vi "Agilent 34970 EZ Scan-AJ Version.vi"() -> ()   [LabVIEW 2018]
doc: "This Example VI shows how to set up the scan list and then take a measurement. This VI uses the EZ measurement VIs. These VIs offer the quickest and easiest use. However, they do not let you have different types of measurements in the same scan list. For a full description of the three ways to setup and scan using the HP34970A, read the text below.\n\nAlthough this driver only shows Current and Frequency (for simplicity), there are EZ Measurement VIs for all six measurement types.\n\n====================\nSetting up and performing a scan\n====================\nThe HP34970A provides commands for setting up a scan in three ways that differ in their complexity and the amount of control offered:\n\n1. Advanced:\nEvery aspect of the measurement, scan, scan list, and read is put in a different command to allow the greatest flexibility. For example, using the advanced configure VIs, you can set up a scan list consisting of different measurement types on different channels. The \"HP34970A Advanced Scan Example.vi\" demonstrates usage of these VIs.\n\n2. Medium:\nThe instrument also offers a command that wraps up configuring individual channels and the scan list. This is represented in the driver by \"HP34970A Conf EZ.vi\". This driver specifically replaces use of the advanced configure measurement VIs and configure scan list VIs. For more information, refer to the context help for the Conf EZ VI.\n\n3. Easiest:\nThe entire configuration, scan, and read are wrapped up into one command to the instrument. This is provided in this driver as the \"EZ\" VIs, which are in the Data subpalette of the HP34970A's driver palette. The \"HP34970A EZ Scan Example.vi\" demonstrates the EZ VI's usage."
uses:
  Agilent 34970.lvlib
panel:
  in  "Thermocouple Type":T1(ring)=enum."Default (Last)"
  in  "Resolution (5:Default)":T2(ring)=enum."Default"
  in  "Range":T3(ring)=enum."Auto"
  in  "AC/DC":bool
  in  "Measurement Type":u16(ring) items=["Current", "Frequency/Period", "Voltage", "Temperature"]
  out "Readings":dbl[](array[numeric]) format="%.2f"
  in  "Range":u16(ring)=3 items=["10 mA", "100 mA", "1 A", "Auto", "Minimum", "Maximum"]
  in  "Freq/Period":bool
  in  "Range":T3(ring)=enum."Auto"
  in  "Serial Port Configuration":T4={"Timeout Value (10000)"=10000, "Baud Rate (57600)"=enum."57600", "Flow Control (1:XON/XOFF)"=enum."XON / XOFF"}
  in  "Reset":bool=TRUE
  in  "AC/DC":bool
  in  "Channel List":string
  in  "VISA resource name":refnum<visa-resource-name>
  # "(c) 2005-2010 National Instruments.  ALL RIGHTS RESERVED."
  # "This Example VI shows how to setup the scan list and then then take a measurement.  This VI uses the EZ measurement VIs.  These VIs offer quick and easy use however do not let you have different types of measurements in the same scan list.  To do this, look at HP34970A Advanced Scan Example.vi.\n\nAlthough this driver only shows Current and Frequency (for simplicity), there are EZ Measurement VIs for all six measurement types."
  # "Current"
  # "Temperature"
  # "Frequency/Period"
  # "Voltage"
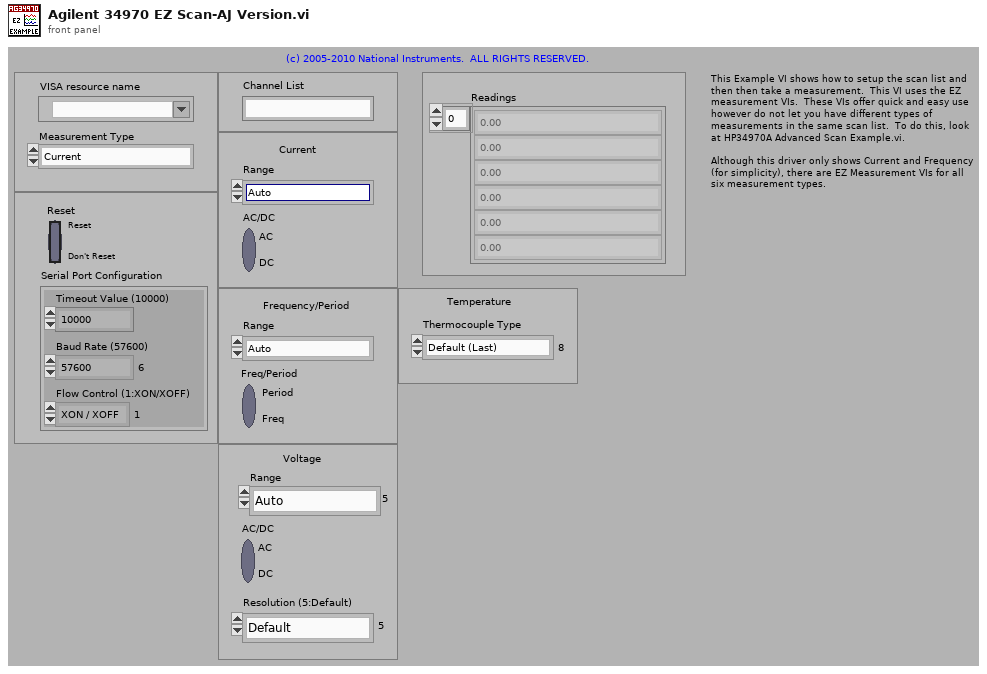
[diagram p1: front panel]
types:
  T1 = enum16{"B", "E", "J", "K", "N", "R", "S", "T", "Default (Last)"}
  T2 = enum16{"4 1/2", "5 1/2", "6 1/2", "Least", "Highest", "Default"}
  T3 = enum16{"100 mV", "1 V", "10 V", "100 V", "300 V", "Auto", "Minimum", "Maximum"}
  T4 = cluster{"Timeout Value (10000)":u32, "Baud Rate (57600)":enum16{"1200", "2400", "4800", "9600", "19200", "38400", "57600", "115200"}, "Flow Control (1:XON/XOFF)":enum16{"None", "XON / XOFF", "RTS / CTS", "DTR / DSR"}}
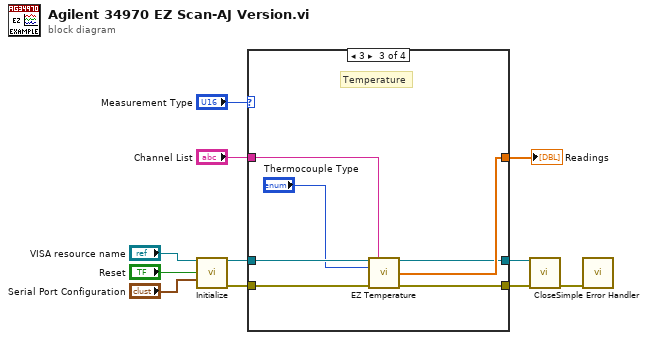
[diagram p0: block diagram]
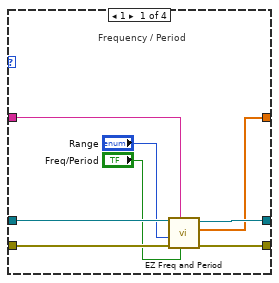
[diagram p2: hidden frame]
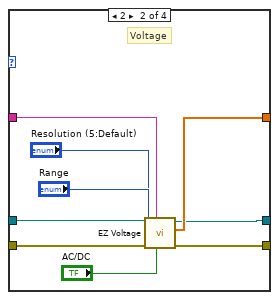
[diagram p3: hidden frame]
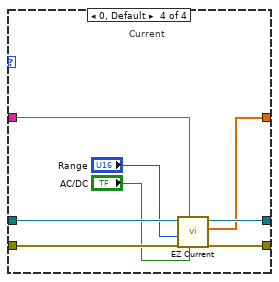
[diagram p4: hidden frame]
diagram:
  n1 = call "Initialize.vi"("VISA Resource Name"="VISA resource name", "Reset (T: Reset)"="Reset", "Serial Port Configuration"="Serial Port Configuration") -> ("VISA Resource Name Out"=w8:refnum<visa-resource-name>, "error out"=w7:errorcluster)  [unwired: 11 in]
  n2 = case shown="3" "Measurement Type" {
    tunnel: w8 -> [w19 w24 w32 w43]
    tunnel: w7 -> [w18 w23 w31 w42]
    tunnel: [w17 w26 w34 w41] -> w5
    tunnel: [w16 w25 w33 w40] -> w4
    tunnel: "Channel List" -> [w13 w28 w30 w37]
    tunnel: [w12 w27 w35 w36] -> w2
    frame 1 {
      # "Frequency / Period"
      n3 = call "EZ Freq and Period.vi"("Freq/Period (F:Freq)"="Freq/Period", "Scan List (empty)"=w13, "error in (no error)"=w18, "Range (5:Auto)"="Range", "VISA Resource Name"=w19) -> ("error out"=w16:errorcluster, "Output Array"=w12:dbl[], "VISA Resource Name Out"=w17:refnum<visa-resource-name>)  [unwired: 4 in]
    }
    frame 2 {
      # "Voltage"
      n4 = call "EZ Voltage.vi"("AC/DC (F:DC)"="AC/DC", "Scan List (empty)"=w28, "error in (no error)"=w23, "Range (5:Auto)"="Range", "Resolution (5:Default)"="Resolution (5:Default)", "VISA Resource Name"=w24) -> ("error out"=w25:errorcluster, "Output Array"=w27:dbl[], "VISA Resource Name Out"=w26:refnum<visa-resource-name>)  [unwired: 3 in]
    }
    frame 3 {
      # "Temperature"
      n5 = call "EZ Temperature.vi"("VISA Resource Name"=w32, "Scan List (empty)"=w30, "Thermocouple Type (8:Def-Last)"="Thermocouple Type", "error in (no error)"=w31) -> ("VISA Resource Name Out"=w34:refnum<visa-resource-name>, "Output Array"=w35:dbl[], "error out"=w33:errorcluster)  [unwired: 9 in]
    }
    frame 0, Default {
      # "Current"
      n6 = call "EZ Current.vi"("DC/AC (F:DC)"="AC/DC", "Scan List (empty)"=w37, "error in (no error)"=w42, "Range (3:Auto)"="Range", "VISA Resource Name"=w43) -> ("error out"=w40:errorcluster, "Output Array"=w36:dbl[], "VISA Resource Name Out"=w41:refnum<visa-resource-name>)  [unwired: 4 in]
    }
  }
  "Readings" <- w2
  n7 = call "Close.vi"("VISA Resource Name"=w5, "error in (no error)"=w4) -> ("error out"=w3:errorcluster)  [unwired: 13 in]
  n8 = call <vilib>:"Simple Error Handler.vi"("error in (no error)"=w3) -> ()  [unwired: 4 in, 5 out]
